vi "Resize window to pane.vi"(7 "Mode":enum16{"Run", "Development"}(ring), 8 "error in":errorcluster, 10 "Splitter Name":string="MainVert", 11 "VI Ref In":refnum<vi>) -> (0 "error out":errorcluster, 3 "VI Ref Out":refnum<vi>)   [LabVIEW 2023]
doc: "This VI allows easy use of front panel real estate for non-UI controls and indicators. Run as part of the window setup when the calling VI is run, and run again to reset the named splitter function to development mode when the VI finishes.\n\nResize window by moving right edge to named splitter (default = \"MainVert\"). Then set that splitter to stick right , so everythign to the left will resize.If refunum in is empty, parent refunum is used."
panel:
  out "Splitter Found":bool
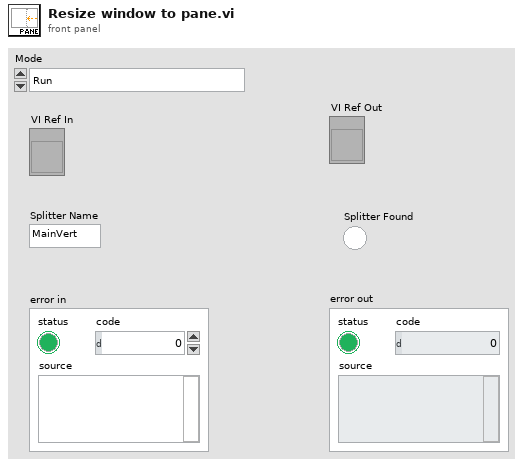
[diagram p1: front panel]
types:
  T1 = enum16{"Sticks Top/Left", "Sticks Bottom/Right", "Proportional"}
  T2 = typedef "LVRectTypeDef.ctl" = cluster{"Left":i16, "Top":i16, "Right":i16, "Bottom":i16}
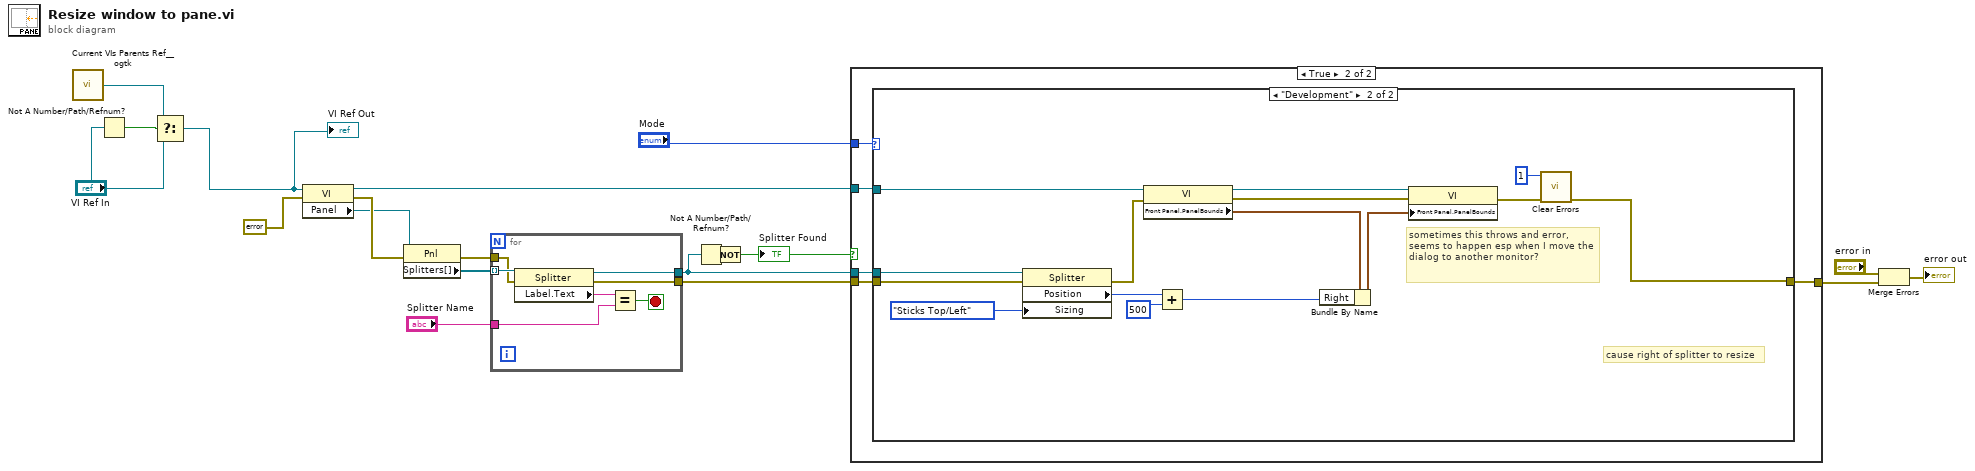
[diagram p0: block diagram]
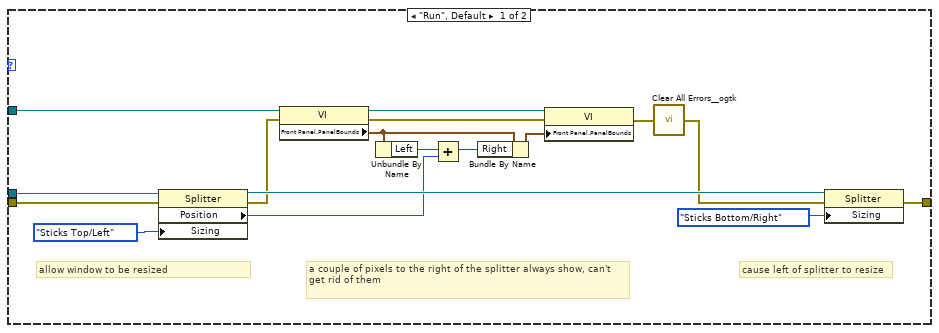
[diagram p3: hidden frame]
diagram:
  n1 = call <userlib>:"Current VIs Parents Ref__ogtk.vi"() -> ("Calling VI's Reference"=w9:refnum<vi>)  [unwired: 2 in]
  n2 = Not A Number/Path/Refnum?(number/path/refnum="VI Ref In") -> (NaN/Path/Refnum?=w10:bool)
  n3 = Select(t=w9, s=w10, f="VI Ref In") -> (s? t:f=w7:refnum<vi>)
  "VI Ref Out" <- w7
  n4 = property class="VI"(reference=w7, error in=errorcluster {"status"=FALSE, "code"=0, "source"=""} ("error in (no error)")) -> (reference out=w12:refnum<vi>, error out=w16:errorcluster, "Panel"=w11:refnum<vi>)
  n5 = property class="Pnl"(reference=w11, error in=w16) -> (error out=w15:errorcluster, "Splitters[]"=w18:refnum<vi>[])  [unwired: 1 out]
  n6 = for {
    tunnel: w18 -> [w26] mode=indexing
    tunnel: [w24] -> w19
    tunnel: "Splitter Name" -> [w23]
    tunnel: w15 -> [w22]
    tunnel: [w21] -> w13
    stop <- w20 stop-if-true
    n7 = property class="Splitter"(reference=w26, error in=w22) -> (reference out=w24:refnum<vi>, error out=w21:errorcluster, "Label.Text"=w25:string)
    n8 = Equal?(x=w25, y=w23) -> (x = y?=w20:bool)
  }
  n9 = Not A Number/Path/Refnum?(number/path/refnum=w19) -> (NaN/Path/Refnum?=w6:bool)
  n10 = Not(x=w6) -> (.not. x?=w5:bool)
  "Splitter Found" <- w5
  n11 = case shown="True" w5 {
    tunnel: w19 -> [_ w32]
    tunnel: "Mode" -> [_ w31]
    tunnel: w13 -> [w27 w30]
    tunnel: w12 -> [_ w29]
    tunnel: [w27 w28] -> w3
    frame False {
    }
    frame True {
      n12 = case shown="\"Development\"" w31 {
        tunnel: [w49 w50] -> w28
        tunnel: w32 -> [w39 w55]
        tunnel: w30 -> [w40 w54]
        tunnel: w29 -> [w38 w52]
        frame "Run", Default {
          # "a couple of pixels to the right of the splitter always show, can't get rid of them"
          # "allow window to be resized"
          # "cause left of splitter to resize"
          n13 = property class="Splitter"(reference=w39, error in=w40, "Sizing"=T1."Sticks Top/Left") -> (reference out=w47:refnum<vi>, error out=w41:errorcluster, "Position"=w33:i32)
          n14 = property class="VI"(reference=w38, error in=w41) -> (reference out=w42:refnum<vi>, error out=w45:errorcluster, "Front Panel.PanelBounds"=w37:T2)
          n15 = Unbundle By Name(w37) -> ("Left"=w36:i16)
          n16 = Add(x=w36, y=w33) -> (x+y=w35:i32)
          n17 = Bundle By Name(cluster=w37, "Right"=w35) -> (w43:T2)
          n18 = property class="VI"(reference=w42, error in=w45, "Front Panel.PanelBounds"=w43) -> (error out=w46:errorcluster)  [unwired: 1 out]
          n19 = call <userlib>:"Clear All Errors__ogtk.vi"("Error In"=w46) -> ("Error Out"=w34:errorcluster)  [unwired: 3 in]
          n20 = property class="Splitter"(reference=w47, error in=w34, "Sizing"=T1."Sticks Bottom/Right") -> (error out=w49:errorcluster)  [unwired: 1 out]
        }
        frame "Development" {
          # "sometimes this throws and error, seems to happen esp when I move the dialog to another monitor?"
          # "cause right of splitter to resize"
          n21 = property class="Splitter"(reference=w55, error in=w54, "Sizing"=T1."Sticks Top/Left") -> (error out=w59:errorcluster, "Position"=w58:i32)  [unwired: 1 out]
          n22 = property class="VI"(reference=w52, error in=w59) -> (reference out=w60:refnum<vi>, error out=w63:errorcluster, "Front Panel.PanelBounds"=w62:T2)
          n23 = Add(x=w58, y=500) -> (x+y=w56:i32)
          n24 = Bundle By Name(cluster=w62, "Right"=w56) -> (w61:T2)
          n25 = property class="VI"(reference=w60, error in=w63, "Front Panel.PanelBounds"=w61) -> (error out=w64:errorcluster)  [unwired: 1 out]
          n26 = call <vilib>:"Clear Errors.vi"("error in (no error)"=w64, "specific error code to clear (0: all)"=1) -> ("error out"=w50:errorcluster)  [unwired: 4 in, 1 out]
        }
      }
    }
  }
  n27 = Merge Errors("error in", w3) -> (→"error out":errorcluster)
